vi "Enable Light Write.vi"(8 "error in (no error)":errorcluster, 9 "Enable Light?":bool, 11 "3D Plot.lvclass in":refnum<class "3D Plot.lvclass">) -> (0 "error out":errorcluster, 3 "3D Plot.lvclass out":refnum<class "3D Plot.lvclass">)   [LabVIEW 2017, in "3D Plot.lvclass"]
uses:
  <vilib>/Math Plots/3D Math Plots/3D Plot/3D Plot/3D Plot.lvclass
  <vilib>/Math Plots/3D Math Plots/3D Plot/3D Plot/3D Plot.lvclass/3D Plot.ctl
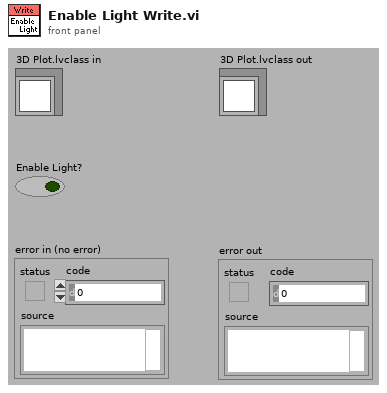
[diagram p1: front panel]
types:
  T1 = typedef "3D Plot.lvclass/Light Specific.ctl" = cluster{"Enable Light?":bool, "Light Color":u32, "Light Latitude":sgl, "Light Longitude":sgl, "Light Distance":sgl, "Attenuation":enum16{"None", "Linear", "Quadratic"}}
  T2 = enum16{"Light 0", "Light 1", "Light 2", "Light 3"}
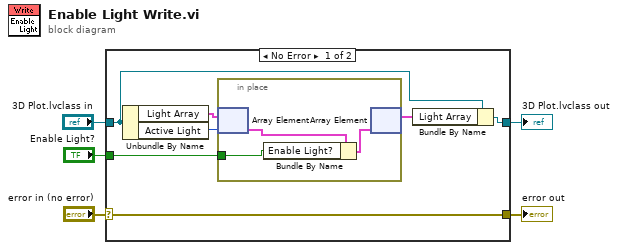
[diagram p0: block diagram]
diagram:
  n1 = case shown="No Error" "error in (no error)" {
    selector: "error in (no error)" -> [w6 w17]
    tunnel: "Enable Light?" -> [w12 _]
    tunnel: "3D Plot.lvclass in" -> [w8 w16]
    tunnel: [w7 w16] -> w3
    tunnel: [w6 w17] -> w1
    frame No Error {
      n2 = Unbundle By Name(w8) -> ("Light Array"=w9:T1[], "Active Light"=w10:T2)
      n3 = in-place {
        in-place-border: w12 -> [w13]
        n4 = in-place-array #1(w9, w10) -> (w15:T1)
        n5 = Bundle By Name(cluster=w15, "Enable Light?"=w13) -> (w14:T1)
        n6 = in-place-array #1(w14) -> (w11:T1[])  [unwired: 1 out]
      }
      n7 = Bundle By Name(cluster=w8, "Light Array"=w11) -> (w7:refnum<class "3D Plot.lvclass">)
    }
    frame Error {
    }
  }
  "error out" <- w1
  "3D Plot.lvclass out" <- w3
